vi "Test parts.vi"() -> ()   [LabVIEW 2015]
panel:
  out "x .xor. y?":cluster{"Device":u16, "Expand":bool}[](array[cluster])
  in  "stop":bool
  in  "Device Array":cluster{"Device":u16, "Expand":bool}[](array[cluster]) {"Device" items=["NONE", "Device 1", "Device 2"]}
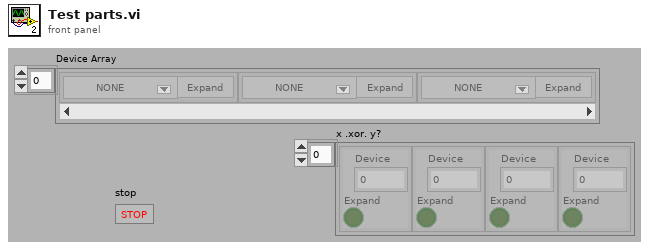
[diagram p1: front panel]
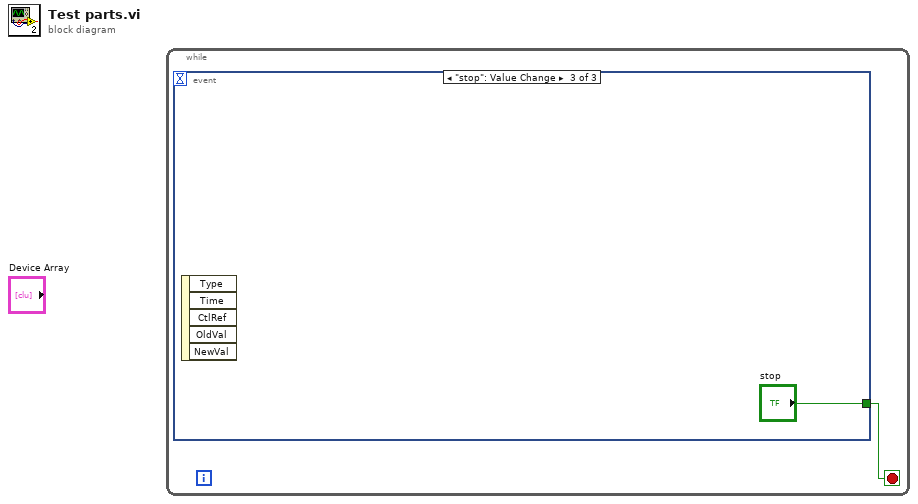
[diagram p0: block diagram]
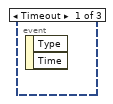
[diagram p2: hidden frame]
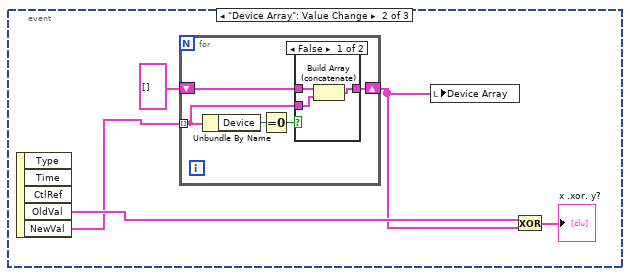
[diagram p3: hidden frame]
diagram:
  n1 = while {
    stop <- w1 stop-if-true
    n2 = event shown="[2] \"stop\": Value Change" {
      selector: _ -> [_ _ _]
      dyn-events: _ -> [_ _ _]
      timeout: _ -> [_ _ _]
      tunnel: [_ _ "stop"] -> w1
      event Timeout {
        n3 = event-data() -> ()  [unwired: 1 in, 2 out]
      }
      event "Device Array": Value Change {
        n4 = event-data() -> ("OldVal"=w6:cluster{"Device":u16, "Expand":bool}[], "NewVal"=w3:cluster{"Device":u16, "Expand":bool}[])  [unwired: 1 in, 3 out]
        n5 = for {
          tunnel: w3 -> [w9] mode=indexing
          shift-right: [w7] -> w2
          shift-left: cluster{"Device":u16, "Expand":bool}[] [] -> [w8]
          n6 = Unbundle By Name(w9) -> ("Device"=w11:u16)
          n7 = Equal To 0?(x=w11) -> (x = 0?=w10:bool)
          n8 = case shown="False" w10 {
            tunnel: w9 -> [w14 _]
            tunnel: [w13 w15] -> w7
            tunnel: w8 -> [w12 w15]
            frame False {
              n9 = Build Array (concatenate)(w12, w14) -> (w13:cluster{"Device":u16, "Expand":bool}[])
            }
            frame True {
            }
          }
        }
        n10 = local write "Device Array"(w2) -> ()
        n11 = Exclusive Or(1:w2, 2:w6) -> (0:→"x .xor. y?":cluster{"Device":u16, "Expand":bool}[])
      }
      event "stop": Value Change {
        n12 = event-data() -> ()  [unwired: 1 in, 5 out]
      }
    }
  }
